vi "CoffeeProcessingPlant.vi"() -> ()   [LabVIEW 2021]
uses:
  <vilib>/numeric/Random Number (Range) U64.vi
  <vilib>/numeric/sub_Random U32.vi
  <vilib>/Utility/file.llb/Write Delimited Spreadsheet (string).vi
panel:
  out "Initial \nSorting\nWeight":dbl
  out "Current \nSorting\nWeight":dbl
  out "Discarded \nSorting\nWeight":dbl
  out "Discarded \nCleaning\nWeight":dbl
  out "Sorting":bool
  out "Discarded Weight":dbl(slide) scale=0.0..600.0
  out "Current Weight":dbl(slide) scale=0.0..600.0
  out "Current \nRoasting\nWeight":dbl
  out "Initial \nRoasting\nWeight":dbl
  out "Current \nRoasting\nMoisture":dbl
  out "Initial \nRoasting\nMoisture":dbl
  out "Current \nDrying\nWeight":dbl
  out "Initial\nDrying\nWeight":dbl
  out "Coffee \nMarket Value":string
  out "Roasting Progress":u8(slide) scale=0.0..100.0
  out "Temperature":dbl(slide) scale=0.0..300.0
  out "Initial \nCleaning\nWeight":dbl
  out "Weight Scale":dbl(knob) scale=0.0..1000.0
  out "Current \nCleaning\nWeight":dbl
  out "Roasting":bool
  out "Initial \nDrying\nMoisture":dbl
  out "Moisture Scale":dbl(knob) scale=0.0..60.0
  out "Current \nDrying\nMoisture":dbl
  out "Cleaning":bool
  out "Drying":bool
  out "Batch Number":dbl
  # "COFFEE PRODUCTION"
  # "DRYING"
  # "CLEANING"
  # "%"
  # "%"
  # "kg"
  # "kg"
  # "kg"
  # "kg"
  # "kg"
  # "ROASTING"
  # "SORTING"
  # "kg"
  # "%"
  # "%"
  # "kg"
  # "kg"
  # "kg"
  # "kg"
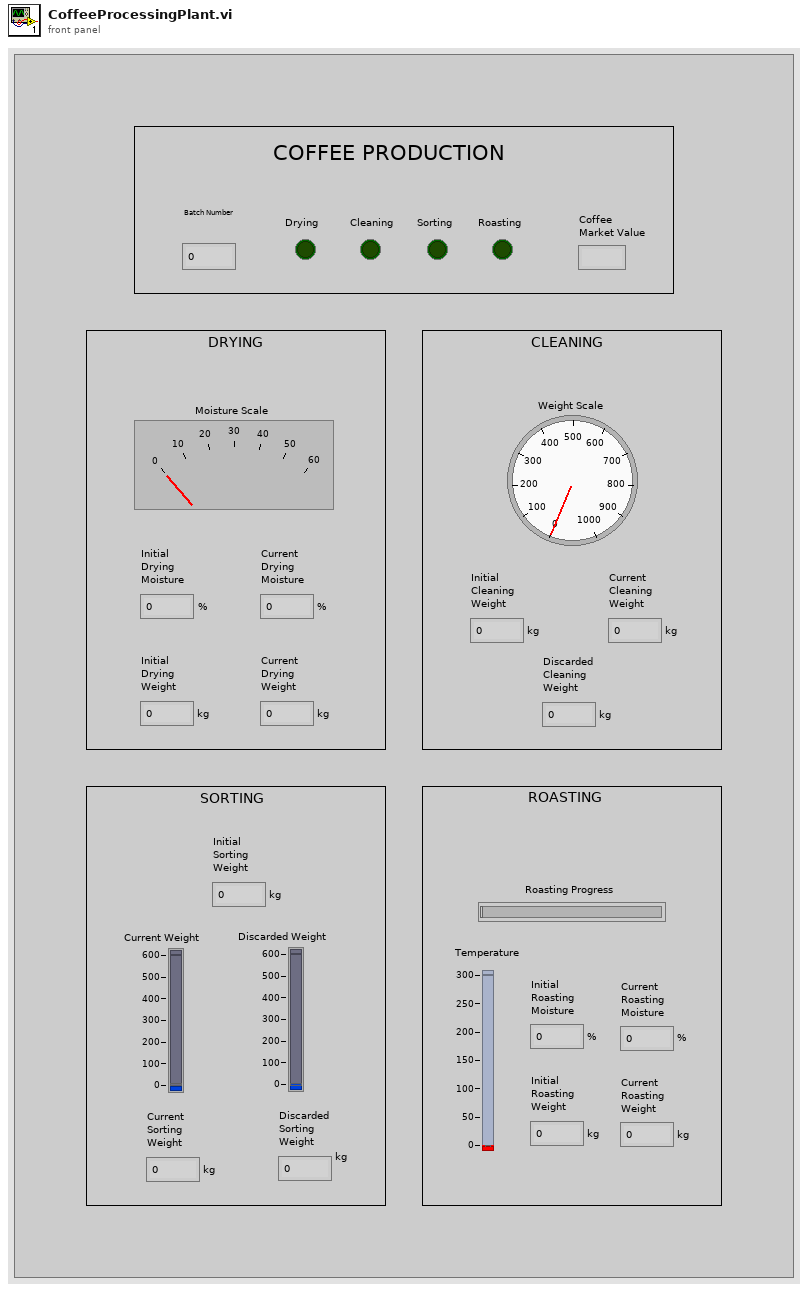
[diagram p1: front panel]
types:
  T1 = enum16{"Read", "Write", "ReadWrite", "BufferedRead", "BufferedReadWrite"}
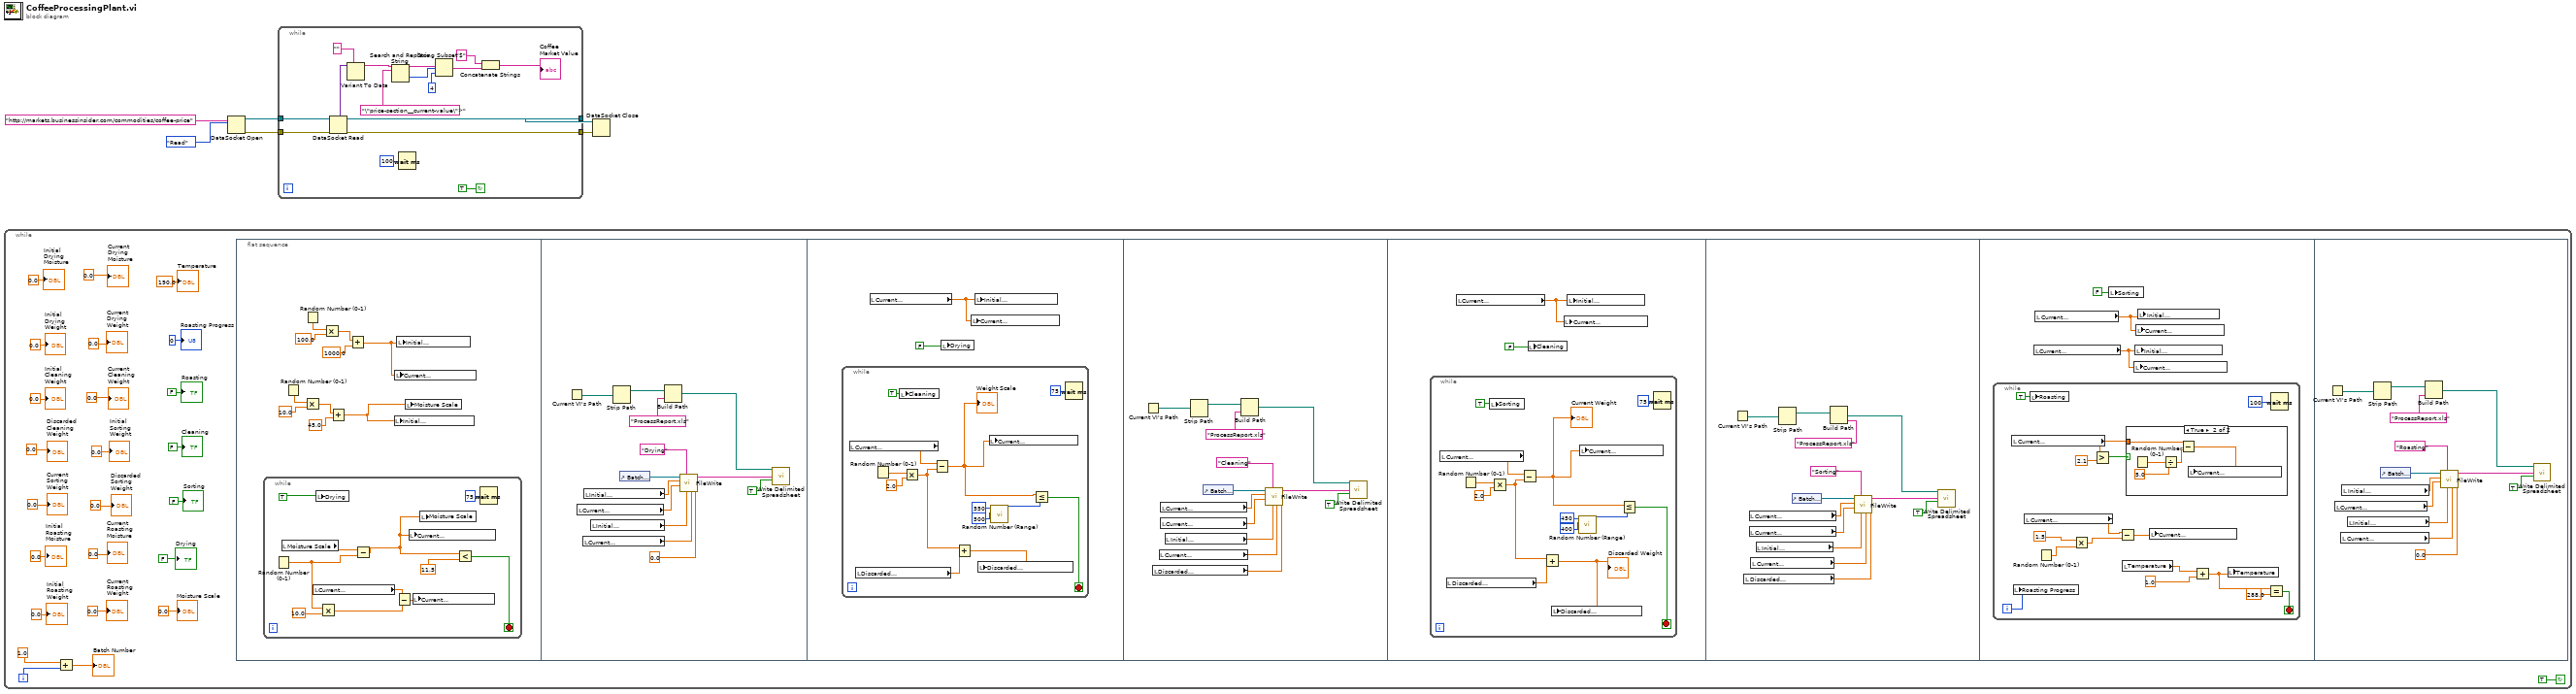
[diagram p0: block diagram]
diagram:
  n1 = while {
    i -> [w13]
    stop <- TRUE continue-if-true
    n2 = Add(x=1.0, y=w13) -> (x+y=→"Batch Number":dbl)
    n3 = flat-sequence {
      frame #0 {
        n4 = while {
          stop <- w48 stop-if-true
          n5 = Random Number (0-1)() -> (number: 0 to 1=w46:dbl)
          n6 = local read "Moisture Scale"() -> (w52:dbl)
          n7 = local read "Current \nDrying\nWeight"() -> (w44:dbl)
          n8 = local write "Drying"(TRUE) -> ()
          n9 = Multiply(x=w46, y=10.0) -> (x*y=w42:dbl)
          n10 = Subtract(x=w52, y=w46) -> (x-y=w47:dbl)
          n11 = Subtract(x=w44, y=w42) -> (x-y=w43:dbl)
          n12 = local write "Current \nDrying\nMoisture"(w47) -> ()
          n13 = local write "Current \nDrying\nWeight"(w43) -> ()
          n14 = local write "Moisture Scale"(w47) -> ()
          n15 = Less?(x=w47, y=11.5) -> (x < y?=w48:bool)
          n16 = Wait (ms)(milliseconds to wait=u32 75) -> ()  [unwired: 1 out]
        }
        n17 = Random Number (0-1)() -> (number: 0 to 1=w40:dbl)
        n18 = Random Number (0-1)() -> (number: 0 to 1=w34:dbl)
        n19 = Multiply(x=w40, y=10.0) -> (x*y=w41:dbl)
        n20 = Multiply(x=w34, y=100.0) -> (x*y=w35:dbl)
        n21 = Add(x=w41, y=45.0) -> (x+y=w37:dbl)
        n22 = Add(x=w35, y=1000.0) -> (x+y=w36:dbl)
        n23 = local write "Initial \nDrying\nMoisture"(w37) -> ()
        n24 = local write "Current \nDrying\nWeight"(w36) -> ()
        n25 = local write "Initial\nDrying\nWeight"(w36) -> ()
        n26 = local write "Moisture Scale"(w37) -> ()
      }
      frame #1 {
        n27 = Current VI's Path() -> (path=w63:path)
        n28 = local read "Current \nDrying\nMoisture"() -> (w59:dbl)
        n29 = local read "Current \nDrying\nWeight"() -> (w57:dbl)
        n30 = local read "Initial \nDrying\nMoisture"() -> (w58:dbl)
        n31 = local read "Initial\nDrying\nWeight"() -> (w60:dbl)
        n32 = Strip Path(path=w63) -> (stripped path=w62:path)  [unwired: 1 out]
        n33 = control-ref of="Batch Number"() -> (w54:refnum<vi>)
        n34 = Build Path(base path=w62, name or relative path="ProcessReport.xls") -> (appended path=w55:path)
        n35 = call "FileWrite"("Discarded\nWeight"=0.0, "Current \nWeight"=w57, "Initial\nWeight"=w60, "element"="Drying", "Current \nMoisture"=w59, "Initial \nMoisture"=w58, "Digital in"=w54) -> ("Array"=w65:string[])  [unwired: 4 in]
        n36 = call-poly <vilib>:"Write Delimited Spreadsheet.vi"("file path (dialog if empty)"=w55, "1D data"=w65, "append to file? (new file:F)"=TRUE) -> ()  [unwired: 11 in, 2 out]
      }
      frame #2 {
        n37 = while {
          stop <- w76 stop-if-true
          n38 = local read "Current \nCleaning\nWeight"() -> (w80:dbl)
          n39 = local read "Discarded \nCleaning\nWeight"() -> (w70:dbl)
          n40 = Random Number (0-1)() -> (number: 0 to 1=w72:dbl)
          n41 = local write "Cleaning"(TRUE ("Sorting")) -> ()
          n42 = Multiply(x=w72, y=2.0 ("x")) -> (x*y=w69:dbl)
          n43 = Subtract(x=w80, y=w69) -> (x-y=w74:dbl)
          "Weight Scale" <- w74
          n44 = Add(x=w69, y=w70) -> (x+y=w68:dbl)
          n45 = local write "Discarded \nCleaning\nWeight"(w68) -> ()
          n46 = local write "Current \nCleaning\nWeight"(w74) -> ()
          n47 = call-poly <vilib>:"Random Number (Range).vi"("lower bound (0)"=u64 500, "upper bound (100)"=u64 550) -> ("number"=w79:u64)  [unwired: 9 in]
          n48 = Less Or Equal?(x=w74, y=w79) -> (x <= y?=w76:bool)
          n49 = Wait (ms)(milliseconds to wait=u32 75) -> ()  [unwired: 1 out]
        }
        n50 = local read "Current \nDrying\nWeight"() -> (w66:dbl)
        n51 = local write "Drying"(FALSE) -> ()
        n52 = local write "Current \nCleaning\nWeight"(w66) -> ()
        n53 = local write "Initial \nCleaning\nWeight"(w66) -> ()
      }
      frame #3 {
        n54 = Current VI's Path() -> (path=w91:path)
        n55 = local read "Discarded \nCleaning\nWeight"() -> (w93:dbl)
        n56 = local read "Current \nCleaning\nWeight"() -> (w86:dbl)
        n57 = local read "Current \nDrying\nMoisture"() -> (w87:dbl)
        n58 = local read "Current \nDrying\nMoisture"() -> (w88:dbl)
        n59 = local read "Initial \nCleaning\nWeight"() -> (w89:dbl)
        n60 = Strip Path(path=w91) -> (stripped path=w90:path)  [unwired: 1 out]
        n61 = control-ref of="Batch Number"() -> (w84:refnum<vi>)
        n62 = Build Path(base path=w90, name or relative path="ProcessReport.xls") -> (appended path=w85:path)
        n63 = call "FileWrite"("Discarded\nWeight"=w93, "Current \nWeight"=w86, "Initial\nWeight"=w89, "element"="Cleaning", "Current \nMoisture"=w88, "Initial \nMoisture"=w87, "Digital in"=w84) -> ("Array"=w92:string[])  [unwired: 4 in]
        n64 = call-poly <vilib>:"Write Delimited Spreadsheet.vi"("file path (dialog if empty)"=w85, "1D data"=w92, "append to file? (new file:F)"=TRUE) -> ()  [unwired: 11 in, 2 out]
      }
      frame #4 {
        n65 = while {
          stop <- w104 stop-if-true
          n66 = local read "Current \nSorting\nWeight"() -> (w108:dbl)
          n67 = local read "Discarded \nSorting\nWeight"() -> (w99:dbl)
          n68 = Random Number (0-1)() -> (number: 0 to 1=w101:dbl)
          n69 = local write "Sorting"(TRUE ("Sorting")) -> ()
          n70 = Multiply(x=w101, y=2.0 ("x")) -> (x*y=w98:dbl)
          n71 = Subtract(x=w108, y=w98) -> (x-y=w97:dbl)
          "Current Weight" <- w97
          n72 = Add(x=w98, y=w99) -> (x+y=w96:dbl)
          "Discarded Weight" <- w96
          n73 = local write "Discarded \nSorting\nWeight"(w96) -> ()
          n74 = call-poly <vilib>:"Random Number (Range).vi"("lower bound (0)"=u64 400, "upper bound (100)"=u64 450) -> ("number"=w107:u64)  [unwired: 9 in]
          n75 = local write "Current \nSorting\nWeight"(w97) -> ()
          n76 = Less Or Equal?(x=w97, y=w107) -> (x <= y?=w104:bool)
          n77 = Wait (ms)(milliseconds to wait=u32 75) -> ()  [unwired: 1 out]
        }
        n78 = local read "Current \nCleaning\nWeight"() -> (w95:dbl)
        n79 = local write "Cleaning"(FALSE) -> ()
        n80 = local write "Current \nSorting\nWeight"(w95) -> ()
        n81 = local write "Initial \nSorting\nWeight"(w95) -> ()
      }
      frame #5 {
        n82 = Current VI's Path() -> (path=w119:path)
        n83 = local read "Discarded \nSorting\nWeight"() -> (w121:dbl)
        n84 = local read "Current \nDrying\nMoisture"() -> (w115:dbl)
        n85 = local read "Current \nDrying\nMoisture"() -> (w116:dbl)
        n86 = local read "Current \nSorting\nWeight"() -> (w114:dbl)
        n87 = local read "Initial \nSorting\nWeight"() -> (w117:dbl)
        n88 = Strip Path(path=w119) -> (stripped path=w118:path)  [unwired: 1 out]
        n89 = control-ref of="Batch Number"() -> (w112:refnum<vi>)
        n90 = Build Path(base path=w118, name or relative path="ProcessReport.xls") -> (appended path=w113:path)
        n91 = call "FileWrite"("Discarded\nWeight"=w121, "Current \nWeight"=w114, "Initial\nWeight"=w117, "element"="Sorting", "Current \nMoisture"=w116, "Initial \nMoisture"=w115, "Digital in"=w112) -> ("Array"=w120:string[])  [unwired: 4 in]
        n92 = call-poly <vilib>:"Write Delimited Spreadsheet.vi"("file path (dialog if empty)"=w113, "1D data"=w120, "append to file? (new file:F)"=TRUE) -> ()  [unwired: 11 in, 2 out]
      }
      frame #6 {
        n93 = while {
          i -> [w138]
          stop <- w135 stop-if-true
          n94 = local read "Current \nRoasting\nMoisture"() -> (w130:dbl)
          n95 = local write "Roasting Progress"(w138) -> ()
          n96 = local read "Current \nRoasting\nWeight"() -> (w128:dbl)
          n97 = local write "Roasting"(TRUE ("Roasting")) -> ()
          n98 = Random Number (0-1)() -> (number: 0 to 1=w126:dbl)
          n99 = Multiply(x=1.5, y=w126) -> (x*y=w127:dbl)
          n100 = Greater?(x=w130, y=2.1) -> (0:w132:bool)
          n101 = Subtract(x=w128, y=w127) -> (x-y=w129:dbl)
          n102 = local read "Temperature"() -> (w140:dbl)
          n103 = case shown="True" w132 {
            tunnel: w130 -> [_ w142]
            frame False {
            }
            frame True {
              n104 = Random Number (0-1)() -> (number: 0 to 1=w144:dbl)
              n105 = Divide(x=w144, y=5.0) -> (x/y=w143:dbl)
              n106 = Subtract(x=w142, y=w143) -> (x-y=w141:dbl)
              n107 = local write "Current \nRoasting\nMoisture"(w141) -> ()
            }
          }
          n108 = local write "Current \nRoasting\nWeight"(w129) -> ()
          n109 = Add(x=w140, y=1.0 ("number (0 to 1)")) -> (x+y=w137:dbl)
          n110 = local write "Temperature"(w137) -> ()
          n111 = Equal?(x=w137, y=288.0) -> (x = y?=w135:bool)
          n112 = Wait (ms)(milliseconds to wait=u32 100 ("millisecond timer value")) -> ()  [unwired: 1 out]
        }
        n113 = local read "Current \nDrying\nMoisture"() -> (w122:dbl)
        n114 = local read "Current \nSorting\nWeight"() -> (w123:dbl)
        n115 = local write "Sorting"(FALSE ("Roasting")) -> ()
        n116 = local write "Current \nRoasting\nMoisture"(w122) -> ()
        n117 = local write "Initial \nRoasting\nMoisture"(w122) -> ()
        n118 = local write "Current \nRoasting\nWeight"(w123) -> ()
        n119 = local write "Initial \nRoasting\nWeight"(w123) -> ()
      }
      frame #7 {
        n120 = Current VI's Path() -> (path=w156:path)
        n121 = local read "Current \nRoasting\nMoisture"() -> (w152:dbl)
        n122 = local read "Current \nRoasting\nWeight"() -> (w150:dbl)
        n123 = local read "Initial \nRoasting\nMoisture"() -> (w151:dbl)
        n124 = local read "Initial \nRoasting\nWeight"() -> (w153:dbl)
        n125 = Strip Path(path=w156) -> (stripped path=w155:path)  [unwired: 1 out]
        n126 = control-ref of="Batch Number"() -> (w147:refnum<vi>)
        n127 = Build Path(base path=w155, name or relative path="ProcessReport.xls") -> (appended path=w148:path)
        n128 = call "FileWrite"("Discarded\nWeight"=0.0, "Current \nWeight"=w150, "Initial\nWeight"=w153, "element"="Roasting", "Current \nMoisture"=w152, "Initial \nMoisture"=w151, "Digital in"=w147) -> ("Array"=w158:string[])  [unwired: 4 in]
        n129 = call-poly <vilib>:"Write Delimited Spreadsheet.vi"("file path (dialog if empty)"=w148, "1D data"=w158, "append to file? (new file:F)"=TRUE) -> ()  [unwired: 11 in, 2 out]
      }
    }
    "Current \nCleaning\nWeight" <- 0.0 ("Current \nSorting\nWeight")
    "Current \nDrying\nMoisture" <- 0.0 ("Current \nDrying\nMoisture")
    "Drying" <- FALSE ("Drying In Process")
    "Moisture Scale" <- 0.0 ("Meter")
    "Initial \nDrying\nMoisture" <- 0.0 ("Initial \nDrying\nMoisture")
    "Initial \nCleaning\nWeight" <- 0.0 ("Initial \nSorting\nWeight")
    "Temperature" <- 190.0 ("Thermometer")
    "Roasting Progress" <- u8 0 ("Slide")
    "Roasting" <- FALSE ("Roasting")
    "Cleaning" <- FALSE ("Sorting")
    "Initial\nDrying\nWeight" <- 0.0 ("Initial\nDrying\nWeight")
    "Current \nDrying\nWeight" <- 0.0 ("Current \nDrying\nWeight")
    "Initial \nRoasting\nWeight" <- 0.0 ("Initial \nRoasting\nWeight")
    "Initial \nRoasting\nMoisture" <- 0.0 ("Initial \nRoasting\nMoisture")
    "Current \nRoasting\nMoisture" <- 0.0 ("Current \nRoasting\nMoisture")
    "Current \nRoasting\nWeight" <- 0.0 ("Current \nRoasting\nWeight")
    "Discarded \nCleaning\nWeight" <- 0.0 ("Initial \nSorting\nMoisture")
    "Initial \nSorting\nWeight" <- 0.0 ("Initial \nSorting\nWeight")
    "Discarded \nSorting\nWeight" <- 0.0 ("Current \nSorting\nMoisture")
    "Current \nSorting\nWeight" <- 0.0 ("Current \nSorting\nWeight")
    "Sorting" <- FALSE ("Sorting")
  }
  n130 = DataSocket Open(10:T1."Read" ("mode"), 11:"http://markets.businessinsider.com/commodities/coffee-price" ("URL")) -> (0:w2:errorcluster, 3:w1:refnum<k13>)  [unwired: 2 in]
  n131 = while {
    tunnel: [w174] -> w6
    tunnel: [w173] -> w5
    tunnel: w2 -> [w168]
    tunnel: w1 -> [w167]
    stop <- TRUE continue-if-true
    n132 = DataSocket Read(8:w168, 11:w167) -> (0:w174:errorcluster, 2:w166:variant, 3:w173:refnum<k13>)  [unwired: 3 in, 4 out]
    n133 = Variant To Data(type="", Variant=w166) -> (data=w164:string)  [unwired: 1 in, 1 out]
    n134 = Search and Replace String(input string=w164, search string="\"price-section__current-value\">") -> (result string=w170:string, offset past replacement=w171:i32)  [unwired: 6 in, 2 out]
    n135 = Wait (ms)(milliseconds to wait=u32 100) -> ()  [unwired: 1 out]
    n136 = String Subset(string=w170, offset (0)=w171, length (rest)=4 ("length (rest)")) -> (substring=w161:string)
    n137 = Concatenate Strings("$" ("string"), w161) -> (→"Coffee \nMarket Value":string)
  }
  n138 = DataSocket Close(8:w6, 11:w5) -> ()  [unwired: 1 in, 2 out]
